vi "InitializeExpectedFrequency.vi"(0 "Interface in":T1, 5 "duration":u32, 11 "error in":errorcluster) -> (4 "Interface out":T1, 15 "error out":errorcluster)   [LabVIEW 2017, in "ThreePhasePLLInterface.lvlib"]
uses:
  ThreePhasePLLInterface.lvlib
  InterfaceRef.ctl
  <instrlib>/_niInstr/Instruction Framework/v1/Host/Instruction Target/niInstr Instruction Target v1 Host.lvclass
  <instrlib>/_niInstr/Instruction Framework/v1/Host/Instruction Framework Context/niInstr Instruction Framework Context v1 Host.lvclass
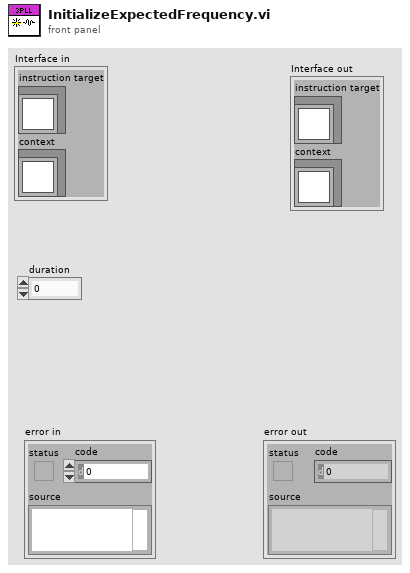
[diagram p1: front panel]
types:
  T1 = typedef "ThreePhasePLLInterface.lvlib/InterfaceRef.ctl" = cluster{"instruction target":refnum<class "niInstr Instruction Target v1 Host.lvclass">, "context":refnum<class "niInstr Instruction Framework Context v1 Host.lvclass">}
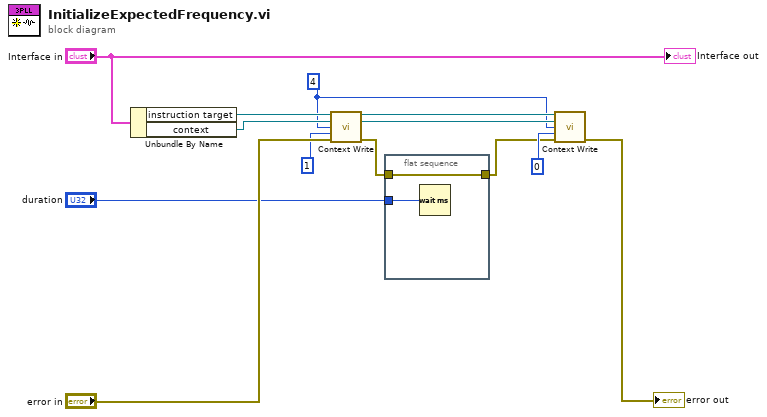
[diagram p0: block diagram]
diagram:
  w6 = u64 4 ("address")
  n1 = Unbundle By Name("Interface in") -> ("instruction target"=w13:refnum<class "niInstr Instruction Target v1 Host.lvclass">, "context"=w12:refnum<class "niInstr Instruction Framework Context v1 Host.lvclass">)
  n2 = call <instrlib>:"Context Write.vi"("instruction target in"=w13, "context in"=w12, "address"=w6, "data"=u64 1, "error in"="error in") -> ("instruction target out"=w8:refnum<class "niInstr Instruction Target v1 Host.lvclass">, "context out"=w7:refnum<class "niInstr Instruction Framework Context v1 Host.lvclass">, "error out"=w3:errorcluster)  [unwired: 8 in]
  n3 = flat-sequence {
    tunnel: w3 -> [w15]
    tunnel: [w15] -> w2
    tunnel: "duration" -> [w14]
    frame #0 {
      n4 = Wait (ms)(milliseconds to wait=w14) -> ()  [unwired: 1 out]
    }
  }
  n5 = call <instrlib>:"Context Write.vi"("instruction target in"=w8, "context in"=w7, "address"=w6, "data"=u64 0, "error in"=w2) -> ("error out"=→"error out":errorcluster)  [unwired: 8 in, 2 out]
  "Interface out" <- "Interface in"
